vi "Add(CSG[]).vi"(1 "Enable(T)":bool=TRUE, 2 "In":csg[](array[numeric]), 4 "n":csg=1.0+0.0i) -> (6 "Out":csg[](array[numeric]) format="%.2f")   [LabVIEW 2013]
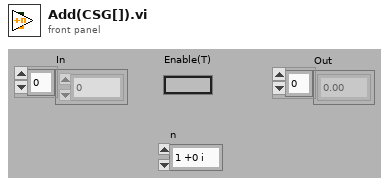
[diagram p1: front panel]
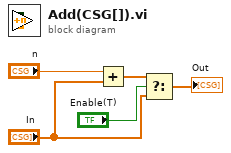
[diagram p0: block diagram]
diagram:
  n1 = Add(x="n", y="In") -> (x+y=w1:csg[])
  n2 = Select(t=w1, s="Enable(T)", f="In") -> (s? t:f=→"Out":csg[])
